vi "Set Modbus Handle.vi"(10 "Modbus Master":refnum<class "Modbus Master.lvclass">, 11 "Island Watch in":refnum<class "Island Watch.lvclass">) -> (3 "Island Watch out":refnum<class "Island Watch.lvclass">)   [LabVIEW 2015, in "Island Watch Actor.lvlib" / "Island Watch.lvclass"]
uses:
  Island Watch.lvclass
  <vilib>/Modbus/master/Modbus Master.lvclass
  Island Watch.lvclass/Island Watch.ctl
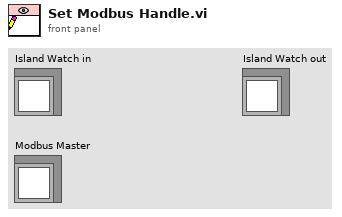
[diagram p1: front panel]
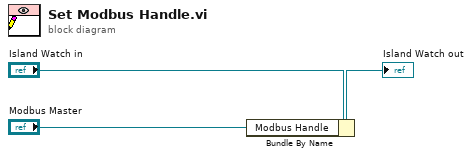
[diagram p0: block diagram]
diagram:
  n1 = Bundle By Name(cluster="Island Watch in", "Modbus Handle"="Modbus Master") -> (→"Island Watch out":refnum<class "Island Watch.lvclass">)
